vi "Maestro_2.vi"() -> ()   [LabVIEW 2017]
uses:
  Enum_1.ctl
  Cluster_Inicial.ctl
  <vilib>/Modbus/master/Modbus Master.lvclass
  <vilib>/Modbus/master/Create Master Instance (TCP).vi
panel:
  out "Conteo 3":bool
  out "Conteo 2":bool
  out "Conteo 1":bool
  out "Conteo":bool
  in  "Ruta del Reporte":path=path "C:/Users/LuisFernando/Documents/UPIITA/8vo semestre/Instrumentacion Virtual Aplicada/Modbus_3"
  in  "stop":bool
  in  "coil values":bool[](array[boolean])
  in  "holding register values":u16[](array[numeric])
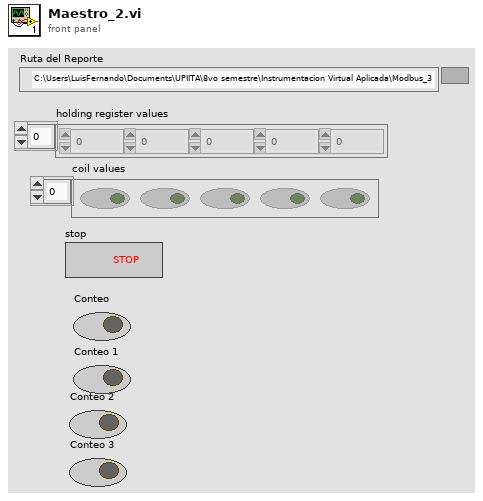
[diagram p1: front panel]
types:
  T1 = typedef "Cluster_Inicial.ctl" = cluster{"TCP master instance":refnum<class "Modbus Master.lvclass">, "error in (no error)":errorcluster, "Ruta del Reporte":path, "Registro":i32, "Conteo del Tiempo":i32, "Registros de Alarmas":i32[], "Numero de Alarma":u32}
  T2 = typedef "Enum_1.ctl" = enum16{"Configuracion", "Espera", "Actualizar Reporte"}
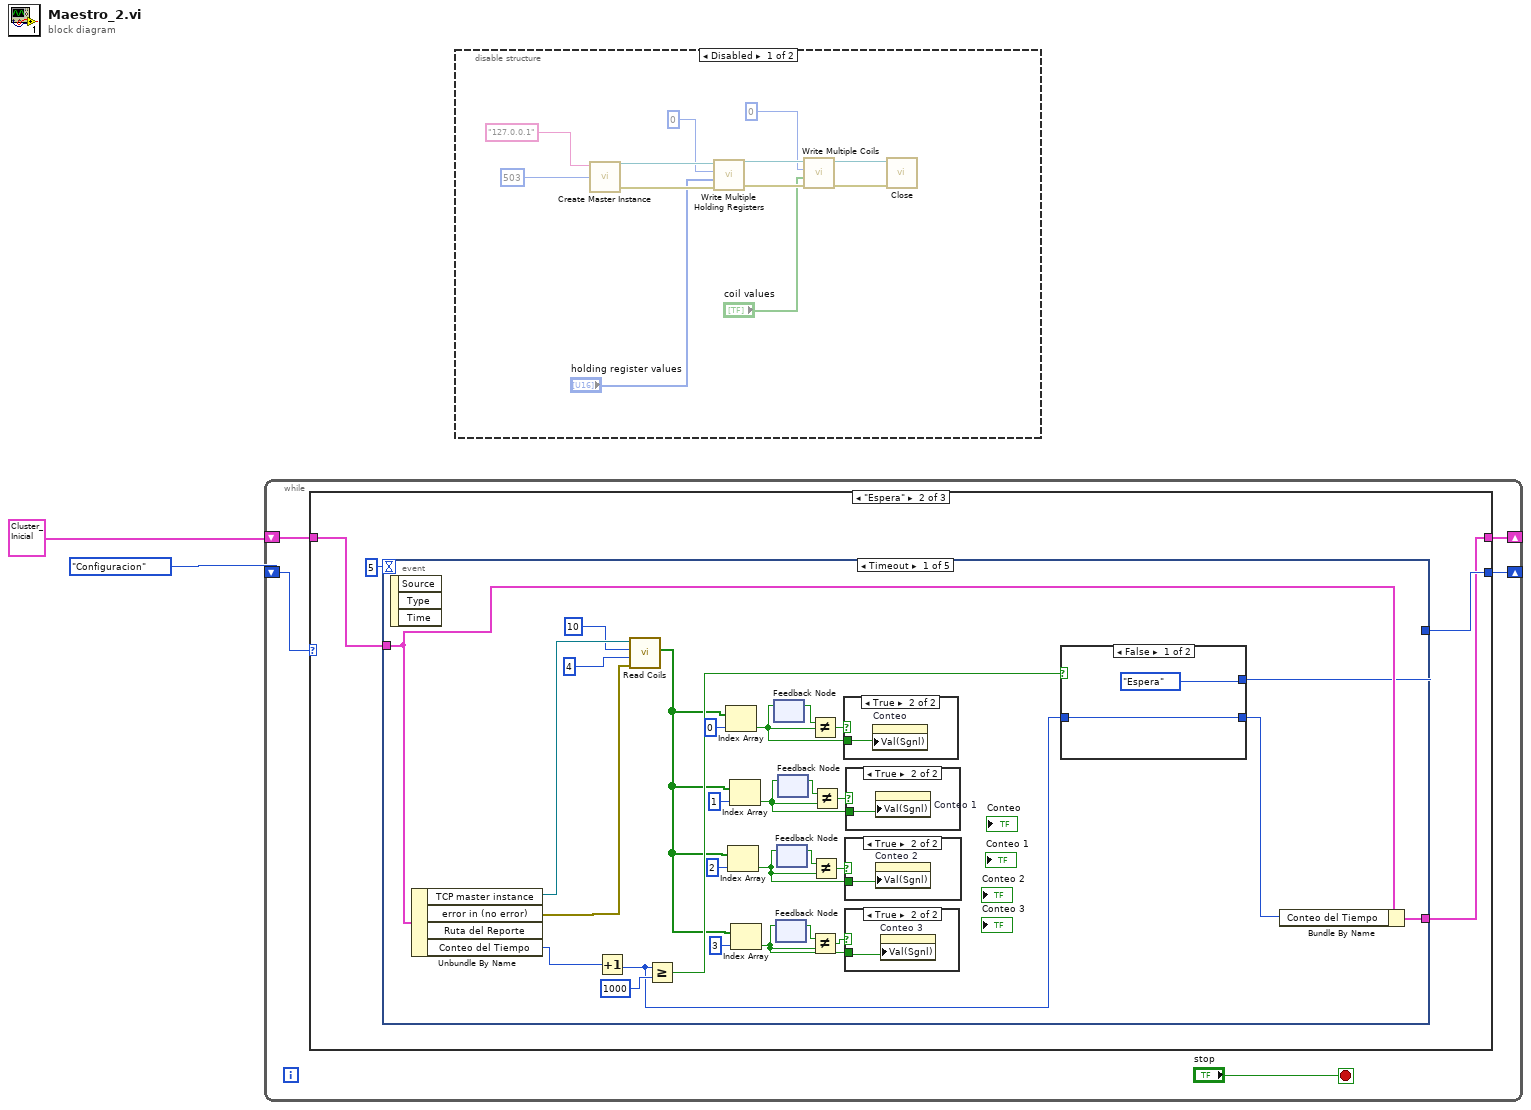
[diagram p0: block diagram]
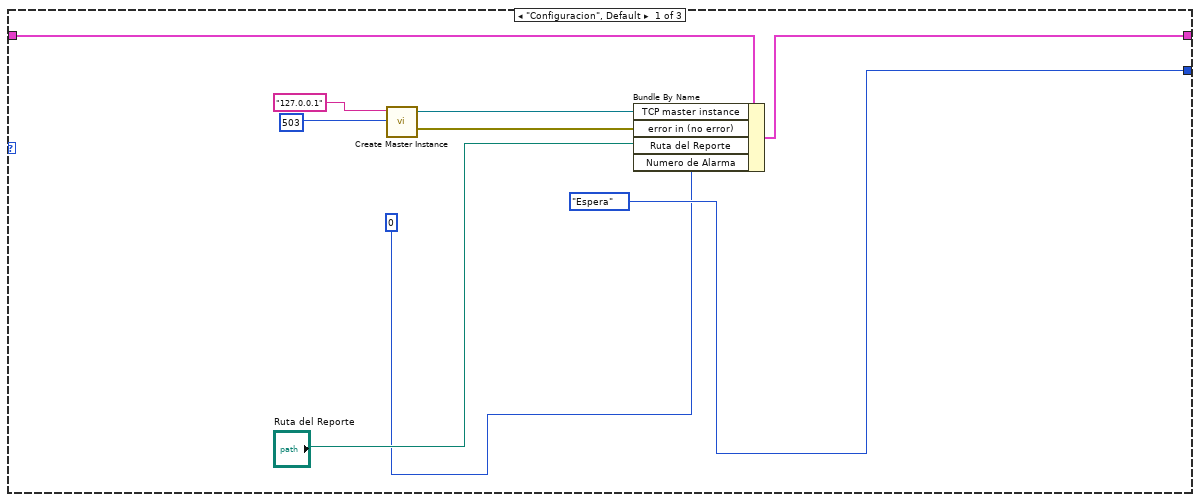
[diagram p2: hidden frame]
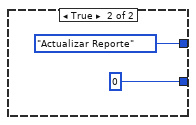
[diagram p7: hidden frame]
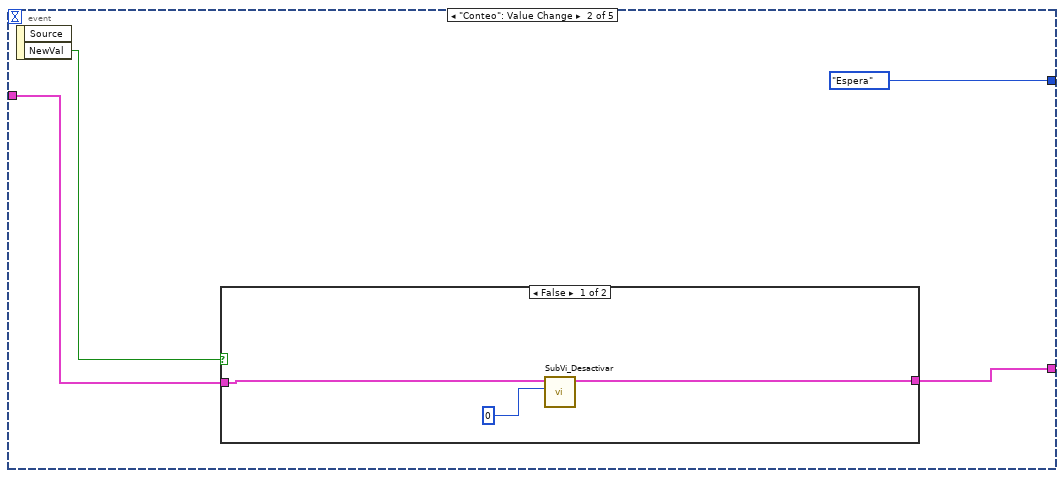
[diagram p8: hidden frame]
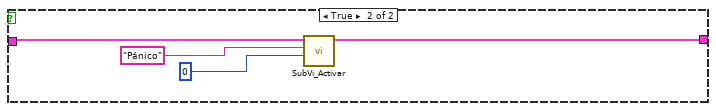
[diagram p9: hidden frame]
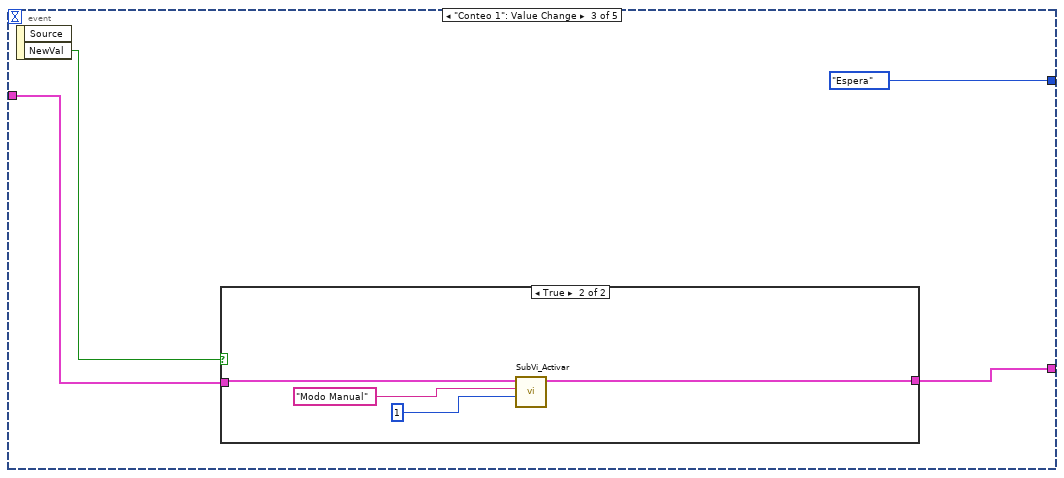
[diagram p10: hidden frame]
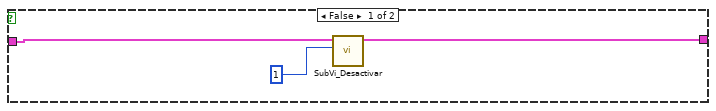
[diagram p11: hidden frame]
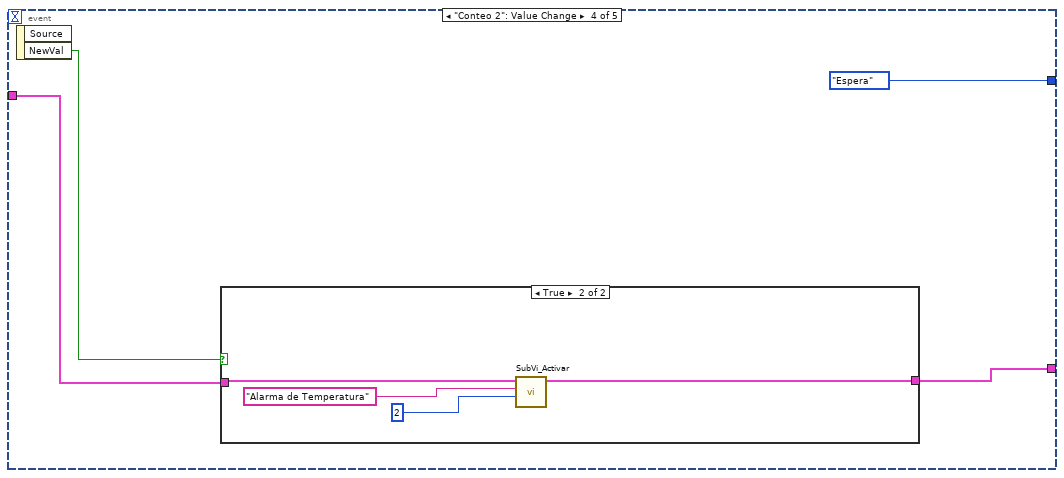
[diagram p12: hidden frame]
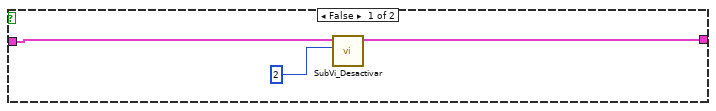
[diagram p13: hidden frame]
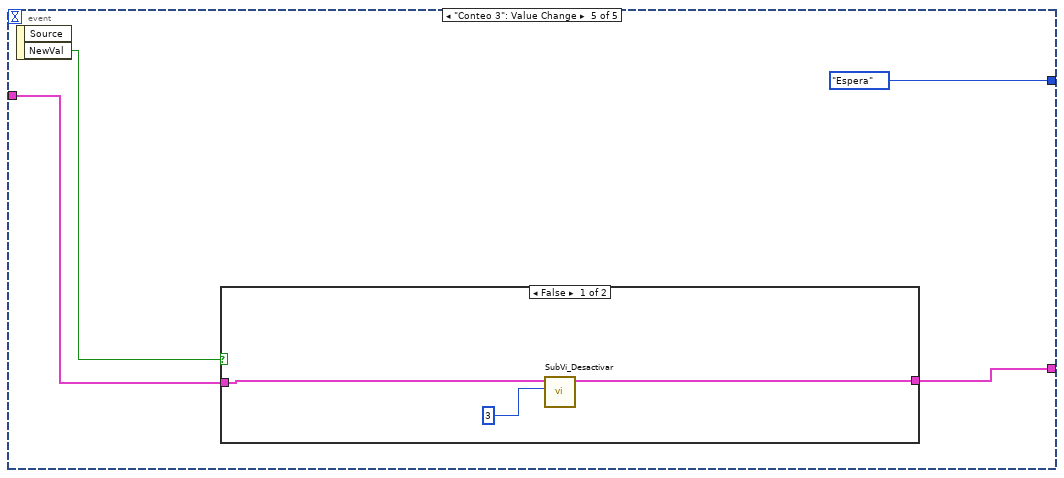
[diagram p14: hidden frame]
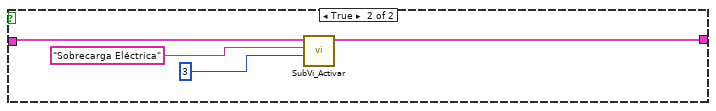
[diagram p15: hidden frame]
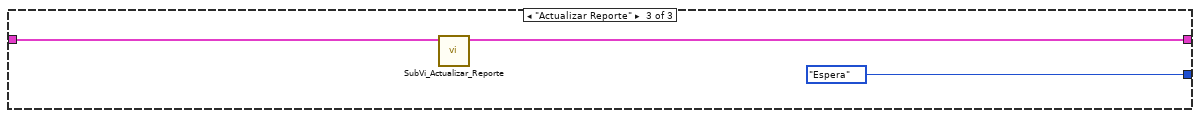
[diagram p16: hidden frame]
diagram:
  n1 = while {
    shift-right: [w3] -> _
    shift-left: Enum_1."Configuracion" -> [w7]
    shift-right: [w5] -> _
    shift-left: T1 {"TCP master instance"=refnum, "error in (no error)"={"status"=FALSE, "code"=0, "source"=""}, "Ruta del Reporte"=path "", "Registro"=0, "Conteo del Tiempo"=0, "Registros de Alarmas"=[0, 0, 0, 0], "Numero de Alarma"=0} ("Cluster out") -> [w6]
    stop <- "stop" stop-if-true
    n2 = case shown="\"Espera\"" w7 {
      tunnel: w6 -> [w14 w19 w103]
      tunnel: [w13 w17 w102] -> w5
      tunnel: [Enum_1."Espera" w18 Enum_1."Espera"] -> w3
      frame "Configuracion", Default {
        n3 = call-poly <vilib>:"Create Master Instance.vi"("port (502)"=u16 503, "address"="127.0.0.1") -> ("error out"=w11:errorcluster, "TCP master instance"=w12:refnum<class "Modbus Master.lvclass">)  [unwired: 8 in]
        n4 = Bundle By Name(cluster=w14, "TCP master instance"=w12, "error in (no error)"=w11, "Ruta del Reporte"="Ruta del Reporte", "Numero de Alarma"=u32 0) -> (w13:T1)
      }
      frame "Espera" {
        n5 = event shown="[0] Timeout" {
          selector: _ -> [_ _ _ _ _]
          dyn-events: _ -> [_ _ _ _ _]
          timeout: 5 -> [_ _ _ _ _]
          tunnel: w19 -> [w42 w60 w71 w82 w93]
          tunnel: [w40 Enum_1."Espera" Enum_1."Espera" Enum_1."Espera" Enum_1."Espera"] -> w18
          tunnel: [w39 w59 w70 w81 w92] -> w17
          event Timeout {
            n6 = event-data() -> ()  [unwired: 1 in, 3 out]
            n7 = Unbundle By Name(w42) -> ("TCP master instance"=w49:refnum<class "Modbus Master.lvclass">, "error in (no error)"=w48:errorcluster, "Conteo del Tiempo"=w45:i32)  [unwired: 1 out]
            n8 = Increment(x=w45) -> (x+1=w38:i32)
            n9 = call-dynamic "Read Coils.vi"("error in (no error)"=w48, "number of coils"=u16 4, "starting address"=u16 10, "Modbus master in"=w49) -> ("coil values"=w25:bool[])  [unwired: 5 in, 2 out]
            n10 = Greater Or Equal?(x=w38, y=1000) -> (x >= y?=w43:bool)
            n11 = Index Array(array=w25, index=0) -> (element=w23:bool)
            n12 = Index Array(array=w25, index=2) -> (element=w22:bool)
            n13 = Index Array(array=w25, index=1) -> (element=w24:bool)
            n14 = Index Array(array=w25, index=3) -> (element=w21:bool)
            n15 = feedback #1() -> (w37:bool)  [unwired: 1 in]
            n16 = feedback-in #1(w23) -> ()
            n17 = feedback #2() -> (w31:bool)  [unwired: 1 in]
            n18 = feedback-in #2(w21) -> ()
            n19 = feedback #3() -> (w33:bool)  [unwired: 1 in]
            n20 = feedback-in #3(w22) -> ()
            n21 = feedback #4() -> (w35:bool)  [unwired: 1 in]
            n22 = feedback-in #4(w24) -> ()
            n23 = Not Equal?(x=w37, y=w23) -> (x != y?=w36:bool)
            n24 = Not Equal?(x=w31, y=w21) -> (x != y?=w30:bool)
            n25 = Not Equal?(x=w33, y=w22) -> (x != y?=w32:bool)
            n26 = Not Equal?(x=w35, y=w24) -> (x != y?=w34:bool)
            n27 = case shown="True" w36 {
              tunnel: w23 -> [_ w53]
              frame False {
              }
              frame True {
                n28 = property on="Conteo" class="Bool (strict)"("Val(Sgnl)"=w53) -> ()  [unwired: 2 in, 2 out]
              }
            }
            n29 = case shown="True" w32 {
              tunnel: w22 -> [_ w51]
              frame False {
              }
              frame True {
                n30 = property on="Conteo 2" class="Bool (strict)"("Val(Sgnl)"=w51) -> ()  [unwired: 2 in, 2 out]
              }
            }
            n31 = case shown="True" w30 {
              tunnel: w21 -> [_ w50]
              frame False {
              }
              frame True {
                n32 = property on="Conteo 3" class="Bool (strict)"("Val(Sgnl)"=w50) -> ()  [unwired: 2 in, 2 out]
              }
            }
            n33 = case shown="True" w34 {
              tunnel: w24 -> [_ w52]
              frame False {
              }
              frame True {
                n34 = property on="Conteo 1" class="Bool (strict)"("Val(Sgnl)"=w52) -> ()  [unwired: 2 in, 2 out]
              }
            }
            n35 = case shown="False" w43 {
              tunnel: [w54 0] -> w41
              tunnel: [Enum_1."Espera" Enum_1."Actualizar Reporte"] -> w40
              tunnel: w38 -> [w54 _]
              frame False {
              }
              frame True {
              }
            }
            n36 = Bundle By Name(cluster=w42, "Conteo del Tiempo"=w41) -> (w39:T1)
          }
          event "Conteo": Value Change {
            n37 = event-data() -> ("NewVal"=w61:bool)  [unwired: 1 in, 1 out]
            n38 = case shown="False" w61 {
              tunnel: w60 -> [w64 w68]
              tunnel: [w62 w65] -> w59
              frame False {
                n39 = call "SubVi_Desactivar.vi"("Indice de Alarma"=0, "input cluster"=w64) -> ("output cluster"=w62:T1)  [unwired: 9 in]
              }
              frame True {
                n40 = call "SubVi_Activar.vi"("Indice de Alarma"=0, "Nombre de Alarma"="Pánico", "input cluster"=w68) -> ("output cluster"=w65:T1)  [unwired: 8 in]
              }
            }
          }
          event "Conteo 1": Value Change {
            n41 = event-data() -> ("NewVal"=w72:bool)  [unwired: 1 in, 1 out]
            n42 = case shown="True" w72 {
              tunnel: w71 -> [w75 w79]
              tunnel: [w73 w76] -> w70
              frame False {
                n43 = call "SubVi_Desactivar.vi"("Indice de Alarma"=1, "input cluster"=w75) -> ("output cluster"=w73:T1)  [unwired: 9 in]
              }
              frame True {
                n44 = call "SubVi_Activar.vi"("Indice de Alarma"=1, "Nombre de Alarma"="Modo Manual", "input cluster"=w79) -> ("output cluster"=w76:T1)  [unwired: 8 in]
              }
            }
          }
          event "Conteo 2": Value Change {
            n45 = event-data() -> ("NewVal"=w83:bool)  [unwired: 1 in, 1 out]
            n46 = case shown="True" w83 {
              tunnel: w82 -> [w86 w90]
              tunnel: [w84 w87] -> w81
              frame False {
                n47 = call "SubVi_Desactivar.vi"("Indice de Alarma"=2, "input cluster"=w86) -> ("output cluster"=w84:T1)  [unwired: 9 in]
              }
              frame True {
                n48 = call "SubVi_Activar.vi"("Indice de Alarma"=2, "Nombre de Alarma"="Alarma de Temperatura", "input cluster"=w90) -> ("output cluster"=w87:T1)  [unwired: 8 in]
              }
            }
          }
          event "Conteo 3": Value Change {
            n49 = event-data() -> ("NewVal"=w94:bool)  [unwired: 1 in, 1 out]
            n50 = case shown="False" w94 {
              tunnel: w93 -> [w97 w101]
              tunnel: [w95 w98] -> w92
              frame False {
                n51 = call "SubVi_Desactivar.vi"("Indice de Alarma"=3, "input cluster"=w97) -> ("output cluster"=w95:T1)  [unwired: 9 in]
              }
              frame True {
                n52 = call "SubVi_Activar.vi"("Indice de Alarma"=3, "Nombre de Alarma"="Sobrecarga Eléctrica", "input cluster"=w101) -> ("output cluster"=w98:T1)  [unwired: 8 in]
              }
            }
          }
        }
      }
      frame "Actualizar Reporte" {
        n53 = call "SubVi_Actualizar_Reporte.vi"("Cluster In"=w103) -> ("Cluster out"=w102:T1)  [unwired: 10 in]
      }
    }
  }
  n54 = disable-structure shown="Disabled" {
    frame Disabled {
      n55 = call-poly <vilib>:"Create Master Instance.vi"("port (502)"=u16 503, "address"="127.0.0.1") -> ("error out"=w115:errorcluster, "TCP master instance"=w116:refnum<class "Modbus Master.lvclass">)  [unwired: 8 in]
      n56 = call-dynamic "Write Multiple Holding Registers.vi"("error in (no error)"=w115, "holding register values"="holding register values", "starting address"=u16 0, "Modbus master in"=w116) -> ("error out"=w109:errorcluster, "Modbus master out"=w110:refnum<class "Modbus Master.lvclass">)  [unwired: 6 in]
      n57 = call-dynamic "Write Multiple Coils.vi"("error in (no error)"=w109, "coil values"="coil values", "starting address"=u16 0, "Modbus master in"=w110) -> ("error out"=w106:errorcluster, "Modbus master out"=w105:refnum<class "Modbus Master.lvclass">)  [unwired: 6 in]
      n58 = call-dynamic "Close.vi"("error in (no error)"=w106, "Modbus master in"=w105) -> ()  [unwired: 9 in, 1 out]
    }
    frame Enabled {
    }
  }
